vi "Force File Move__ogtk.vi"(4 "error in (no error)":errorcluster, 5 "maintain original rights (T)":bool=TRUE, 6 "source":path, 7 "target":path) -> (0 "error out":errorcluster, 3 "target out":path)   [LabVIEW 2014, in "ZLIB.lvlib"]
doc: "Moves a file, forcing it even if the target does already exist and/or is write protected."
uses:
  ZLIB.lvlib
panel:
  # "Force File Move.vi\n\nMoves a file, forcing it even if the target does already exist and/or is write protected.\n\nPlease visit http://www.OpenG.org to learn about the\nOpen Source LabVIEW software movement.\n\nNOTICE -- YOU MUST LEAVE THIS NOTICE IN PLACE.  PER THE TERMS OF THE LICENSE BELOW, YOU MAY SUBLICENSE THIS SOFTWARE \nIN ANY WAY THAT DOES NOT CONFLICT WITH THIS LICENSE.\n\n### BSD License (http://www.opensource.org/licenses/bsd-license.php) Begin ###\n\nCopyright (c) 2004, Rolf Kalbermatter <rolf.kalbermatter@citeng.com>\nCopyright (c) 2006, Jim Kring <jim@jimkring.com>\n\nAll rights reserved.\n\nRedistribution and use in source and binary forms, with or without modification, are permitted provided that the following conditions are met:\n\n    * Redistributions of source code must retain the above copyright notice, this list of conditions and the following disclaimer.\n    * Redistributions in binary form must reproduce the above copyright notice, this list of conditions and the following disclaimer in the \n       documentation and/or other materials provided with the distribution.\n    * Neither the name of SciWare, James Kring, Inc., nor the names of its contributors may be used to endorse or promote products derived \n       from this software without specific prior written permission.\n\nTHIS SOFTWARE IS PROVIDED BY THE COPYRIGHT HOLDERS AND CONTRIBUTORS \"AS IS\" AND ANY EXPRESS OR IMPLIED WARRANTIES, \nINCLUDING, BUT NOT LIMITED TO, THE IMPLIED WARRANTIES OF MERCHANTABILITY AND FITNESS FOR A PARTICULAR PURPOSE ARE \nDISCLAIMED. IN NO EVENT SHALL THE COPYRIGHT OWNER OR CONTRIBUTORS BE LIABLE FOR ANY DIRECT, INDIRECT, INCIDENTAL,\n SPECIAL, EXEMPLARY, OR CONSEQUENTIAL DAMAGES (INCLUDING, BUT NOT LIMITED TO, PROCUREMENT OF SUBSTITUTE GOODS OR \nSERVICES; LOSS OF USE, DATA, OR PROFITS; OR BUSINESS INTERRUPTION) HOWEVER CAUSED AND ON ANY THEORY OF LIABILITY, \nWHETHER IN CONTRACT, STRICT LIABILITY, OR TORT (INCLUDING NEGLIGENCE OR OTHERWISE) ARISING IN ANY WAY OUT OF THE USE \nOF THIS SOFTWARE, EVEN IF ADVISED OF THE POSSIBILITY OF SUCH DAMAGE.\n\n### BSD License End ###"
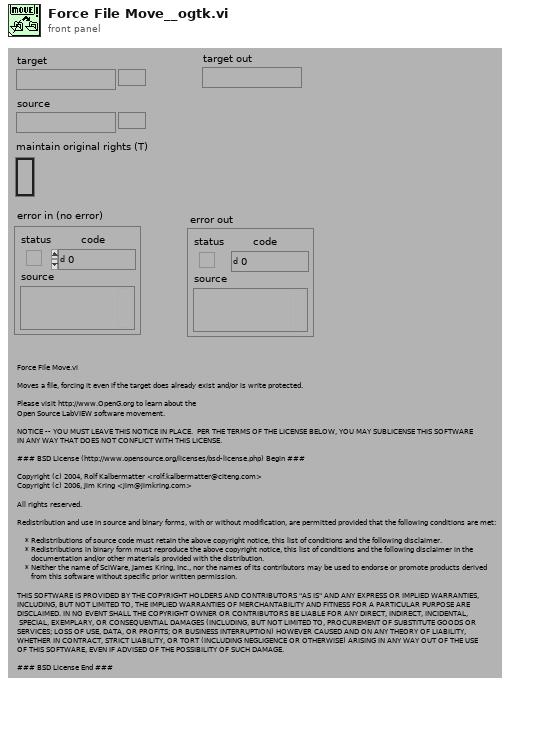
[diagram p1: front panel]
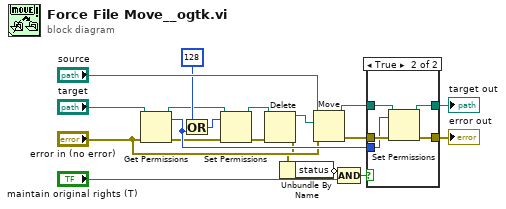
[diagram p0: block diagram]
diagram:
  n1 = Get Permissions(8:"error in (no error)", 11:"target") -> (0:w10:errorcluster, 3:w8:path, 5:w12:i16)  [unwired: 2 out]
  n2 = Or(x=i16 128 ("new permissions"), y=w12) -> (x .or. y?=w11:i16)
  n3 = Set Permissions(7:w11, 8:w10, 11:w8) -> (0:w9:errorcluster, 3:w7:path)  [unwired: 2 in]
  n4 = Delete(path (use dialog)=w7, error in=w9) -> (deleted path=w14:path, error out=w4:errorcluster)  [unwired: 3 in, 1 out]
  n5 = Unbundle By Name(w4) -> ("status"=w3:bool)
  n6 = Move(source path="source", error in="error in (no error)", 10:w14) -> (error out=w17:errorcluster, 3:w15:path)  [unwired: 2 in, 1 out]
  n7 = Compound Arithmetic op=AND(invert w3, "maintain original rights (T)") -> (w1:bool)
  n8 = case shown="True" w1 {
    tunnel: w17 -> [w20 w26]
    tunnel: [w20 w25] -> w16
    tunnel: w15 -> [w21 w24]
    tunnel: w12 -> [_ w23]
    tunnel: [w21 w22] -> w6
    frame False {
    }
    frame True {
      n9 = Set Permissions(7:w23, 8:w26, 11:w24) -> (0:w25:errorcluster, 3:w22:path)  [unwired: 2 in]
    }
  }
  "error out" <- w16
  "target out" <- w6
